vi "tlc_Shutdown.vi"(8 "error in (no error)":errorcluster) -> (0 "error out":errorcluster)   [LabVIEW 2009]
doc: "[Covers: REQ_Close]\nThis VI closes the application safely."
uses:
  Controls/tlc_User Interface Data Type.ctl
  Modules/Display/tlc_Display_Command Control.ctl
  Modules/Hardware/tlc_Hardware_Command Control.ctl
  Modules/File/tlc_File_Command Control.ctl
  Modules/Cue/tlc_Cue_Information Command.ctl
panel:
  # "Input"
  # "Output"
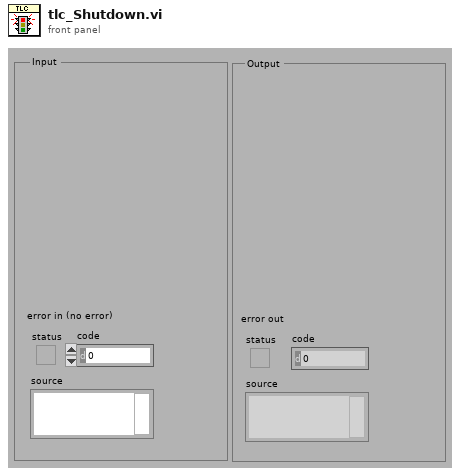
[diagram p1: front panel]
types:
  T1 = typedef "tlc_Cue_Information Command.ctl" = enum16{"Add Cue", "Get Cue Values", "Set Cue Values", "Get Number of Cues", "Initialize", "Get Empty Cue"}
  T2 = typedef "tlc_File_Command Control.ctl" = enum16{"Initialize", "Save Cues", "Load Cues", "Shutdown"}
  T3 = typedef "tlc_Hardware_Command Control.ctl" = enum16{"Initialize", "Write", "Shutdown"}
  T4 = typedef "tlc_Display_Command Control.ctl" = enum16{"Initialize", "Update UI", "Shutdown"}
  T5 = typedef "tlc_User Interface Data Type.ctl" = enum16{"Initialize", "Initialize Front Panel", "Update Front Panel Channels", "Select Cue in Cue List", "Enable/Disable Front Panel Controls", "Update Cue List", "Stop"}
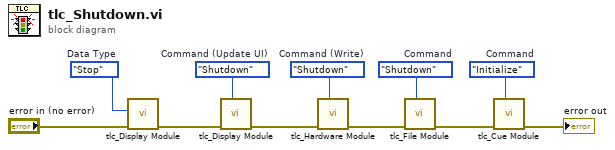
[diagram p0: block diagram]
diagram:
  w1 = tlc_Cue_Information_Command."Initialize"  # Command
  w2 = tlc_File_Command_Control."Shutdown"  # Command
  w7 = tlc_Hardware_Command_Control."Shutdown"  # Command (Write)
  w8 = tlc_Display_Command_Control."Shutdown"  # Command (Update UI)
  w11 = tlc_User_Interface_Data_Type."Stop"  # Data Type
  n1 = call "tlc_Display Module.vi"("error in (no error)"="error in (no error)", "Data Type"=w11) -> ("error out"=w9:errorcluster)  [unwired: 9 in]
  n2 = call "tlc_Display Module.vi"("Command (Update UI)"=w8, "error in (no error)"=w9) -> ("error out"=w6:errorcluster)  [unwired: 9 in]
  n3 = call "tlc_Hardware Module.vi"("Command (Write)"=w7, "error in (no error)"=w6) -> ("error out"=w5:errorcluster)  [unwired: 9 in]
  n4 = call "tlc_File Module.vi"("Command"=w2, "error in (no error)"=w5) -> ("error out"=w4:errorcluster)  [unwired: 8 in, 1 out]
  n5 = call "tlc_Cue Module.vi"("Command"=w1, "error in (no error)"=w4) -> ("error out"=→"error out":errorcluster)  [unwired: 6 in, 2 out]
